vi "Set Endianness.vi"(6 "Endianness":enum16{"BE", "LE", "unknown"}(ring), 8 "error in (no error)":errorcluster, 11 "Encoding in":refnum<class "CConfig UCS-16 Encoding.lvclass">) -> (0 "error out":errorcluster, 3 "Encoding out":refnum<class "CConfig UCS-16 Encoding.lvclass">)   [LabVIEW 2013, in "CConfig UCS-16 Encoding.lvclass"]
doc: "Copyright 2018, Carya Automatisering, Wiebe Walstra."
uses:
  CConfig UCS-16 Encoding.lvclass
  CConfig UCS-16 Encoding.lvclass/CConfig UCS-16 Encoding.ctl
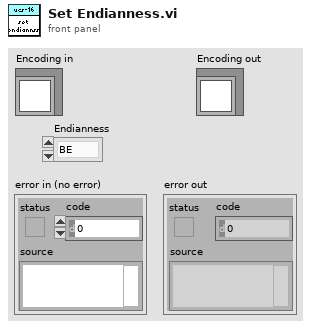
[diagram p1: front panel]
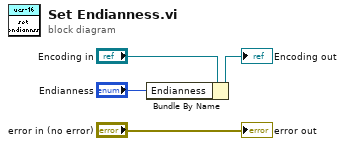
[diagram p0: block diagram]
diagram:
  n1 = Bundle By Name(cluster="Encoding in", "Endianness"="Endianness") -> (→"Encoding out":refnum<class "CConfig UCS-16 Encoding.lvclass">)
  "error out" <- "error in (no error)"
